vi "Import VI Snippet Example.vi"() -> ()   [LabVIEW 2019]
doc: "Example VI to import a VI Snippet (*.png) programmatically into a new VI.\n\nCreated by: Ryan Pacini"
uses:
  <vilib>/Utility/miscctls.llb/LVPositionTypeDef.ctl
panel:
  out "error out":errorcluster
  # "See block diagram for instructions"
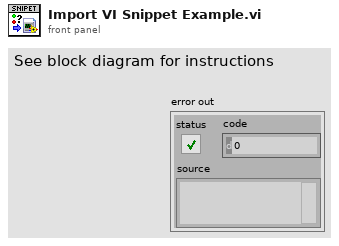
[diagram p1: front panel]
types:
  T1 = typedef "LVPositionTypeDef.ctl" = cluster{"Left":i32, "Top":i32}
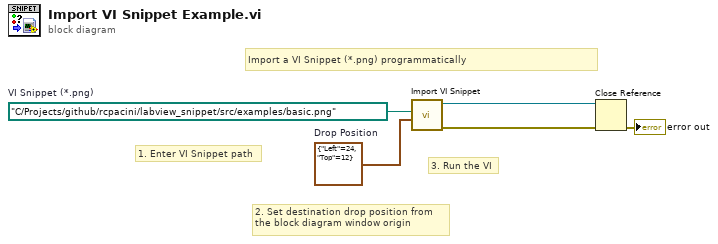
[diagram p0: block diagram]
diagram:
  w4 = T1 {"Left"=24, "Top"=12}  # Drop Position
  w5 = path "C:/Projects/github/rcpacini/labview_snippet/src/examples/basic.png"  # VI Snippet (*.png)
  # "3. Run the VI"
  # "2. Set destination drop position from\nthe block diagram window origin"
  # "1. Enter VI Snippet path"
  # "Import a VI Snippet (*.png) programmatically"
  n1 = call "Import VI Snippet.vi"("Drop Position"=w4, "VI Snippet (*.png)"=w5) -> ("error out"=w3:errorcluster, "VI Refnum out"=w1:refnum<vi>)  [unwired: 7 in, 1 out]
  n2 = Close Reference(reference=w1, error in (no error)=w3) -> (error out=→"error out":errorcluster)
